vi "niDTS BT INSTR RX Configure.vi"(6 "Ports":string[](array[string]), 8 "error in (no error)":errorcluster, 11 "niDTS BT INSTR RX in":refnum<class "niDTS BT INSTR RX.lvclass">) -> (0 "error out":errorcluster, 3 "niDTS BT INSTR RX out":refnum<class "niDTS BT INSTR RX.lvclass">)   [LabVIEW 2015, in "niDTS BT.lvlib" / "niDTS BT INSTR RX.lvclass"]
uses:
  niDTS BT INSTR RX.lvclass
  niDTS BT INSTR RX.lvclass/niDTS BT INSTR RX.ctl
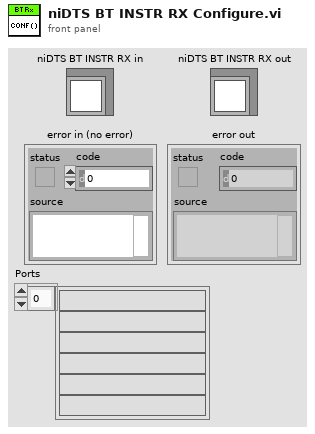
[diagram p1: front panel]
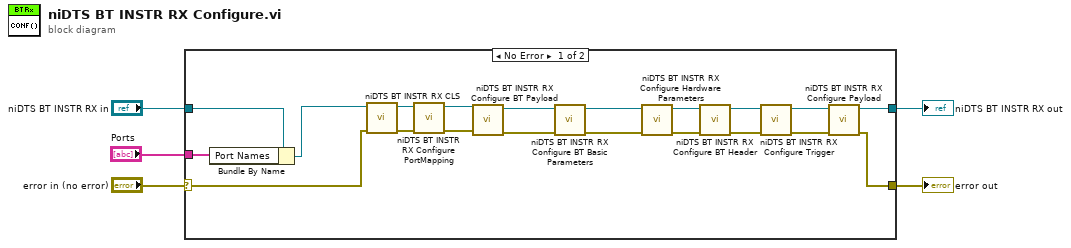
[diagram p0: block diagram]
diagram:
  n1 = case shown="No Error" "error in (no error)" {
    selector: "error in (no error)" -> [w6 w27]
    tunnel: [w16 w27] -> w4
    tunnel: [w14 w26] -> w2
    tunnel: "niDTS BT INSTR RX in" -> [w11 w26]
    tunnel: "Ports" -> [w10 _]
    frame No Error {
      n2 = Bundle By Name(cluster=w11, "Port Names"=w10) -> (w7:refnum<class "niDTS BT INSTR RX.lvclass">)
      n3 = call "niDTS BT INSTR RX CLS.vi"("error in (no error)"=w6, "niDTS BT INSTR RX in"=w7) -> ("error out"=w8:errorcluster, "niDTS BT INSTR RX out"=w9:refnum<class "niDTS BT INSTR RX.lvclass">)  [unwired: 8 in]
      n4 = call "niDTS BT INSTR RX Configure PortMapping.vi"("error in (no error)"=w8, "niDTS BT INSTR RX in"=w9) -> ("error out"=w12:errorcluster, "niDTS BT INSTR RX out"=w13:refnum<class "niDTS BT INSTR RX.lvclass">)  [unwired: 8 in]
      n5 = call-dynamic "niDTS BT INSTR RX Configure BT Payload.vi"("error in (no error)"=w12, "niDTS BT INSTR RX in"=w13) -> ("error out"=w21:errorcluster, "niDTS BT INSTR RX out"=w24:refnum<class "niDTS BT INSTR RX.lvclass">)  [unwired: 8 in]
      n6 = call "niDTS BT INSTR RX Configure BT Basic Parameters.vi"("error in (no error)"=w21, "niDTS BT INSTR RX in"=w24) -> ("error out"=w20:errorcluster, "niDTS BT INSTR RX out"=w25:refnum<class "niDTS BT INSTR RX.lvclass">)  [unwired: 8 in]
      n7 = call "niDTS BT INSTR RX Configure Hardware Parameters.vi"("error in (no error)"=w20, "niDTS BT INSTR RX in"=w25) -> ("error out"=w19:errorcluster, "niDTS BT INSTR RX out"=w23:refnum<class "niDTS BT INSTR RX.lvclass">)  [unwired: 8 in]
      n8 = call "niDTS BT INSTR RX Configure BT Header.vi"("error in (no error)"=w19, "niDTS BT INSTR RX in"=w23) -> ("error out"=w18:errorcluster, "niDTS BT INSTR RX out"=w22:refnum<class "niDTS BT INSTR RX.lvclass">)  [unwired: 8 in]
      n9 = call-dynamic "niDTS BT INSTR RX Configure Trigger.vi"("error in (no error)"=w18, "niDTS BT INSTR RX in"=w22) -> ("error out"=w17:errorcluster, "niDTS BT INSTR RX out"=w15:refnum<class "niDTS BT INSTR RX.lvclass">)  [unwired: 8 in]
      n10 = call-dynamic "niDTS BT INSTR RX Configure Payload.vi"("error in (no error)"=w17, "niDTS BT INSTR RX in"=w15) -> ("error out"=w16:errorcluster, "niDTS BT INSTR RX out"=w14:refnum<class "niDTS BT INSTR RX.lvclass">)  [unwired: 8 in]
    }
    frame Error {
    }
  }
  "error out" <- w4
  "niDTS BT INSTR RX out" <- w2
